vi "Teleop.vi"(10 "Match Info":T1={"Autonomous Elapsed Seconds"=0.0, "TeleOp Elapsed Seconds"=0.0, "Disabled Elapsed Seconds"=0.0, "Visited Autonomous"=FALSE, "Visited TeleOp"=FALSE, "Visited Disabled"=FALSE, "Autonomous Settings"={"Autonomous Style"=enum."Independent", "VI Refnum"=refnum}}, 11 "Call Context":T2) -> ()   [LabVIEW 2013]
doc: "This VI is called for each TeleOp packet received from the DS where the robot is not disabled. It is often used to read from the joysticks and update I/O or to update setpoints for timed control loops. It should complete and return within 20 milliseconds or it may miss DS packets."
uses:
  <vilib>/Rock Robotics/WPI/DriverStation/WPI_DriverStationDerivedRobotMode.ctl
  <vilib>/Rock Robotics/WPI/DriverStation/WPI_DriverStationMatch Info.ctl
  <vilib>/Rock Robotics/WPI/Solenoid/WPI_SolenoidValue.ctl
  Robot Global Data.vi
  <vilib>/Rock Robotics/WPI/Solenoid/Deprecated/WPI_SolenoidGetBool.vi
  <vilib>/Rock Robotics/WPI/Solenoid/WPI_SolenoidSetEnum.vi
  <vilib>/Rock Robotics/WPI/Joystick/WPI_JoystickGetSetRefNum.vi
  <vilib>/Rock Robotics/WPI/RobotDrive/WPI_RobotDriveGetSetRefNum.vi
panel:
  out "Numeric 1":dbl(slide) scale=0.0..100.0
  out "Boolean 2":bool
  out "Boolean 1":bool
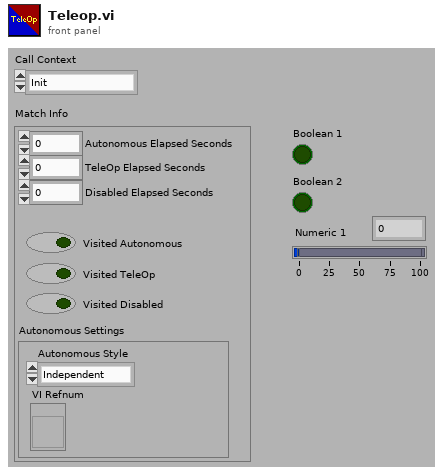
[diagram p1: front panel]
types:
  T1 = typedef "WPI_DriverStationMatch Info.ctl" = cluster{"Autonomous Elapsed Seconds":dbl, "TeleOp Elapsed Seconds":dbl, "Disabled Elapsed Seconds":dbl, "Visited Autonomous":bool, "Visited TeleOp":bool, "Visited Disabled":bool, "Autonomous Settings":cluster{"Autonomous Style":enum16{"Iterative", "Independent"}, "VI Refnum":refnum<vi>}}
  T2 = typedef "WPI_DriverStationDerivedRobotMode.ctl" = enum16{"Init", "Execute", "Stop"}
  T3 = typedef "WPI_JoystickDevRef.ctl" = cluster{"Device":T4}
  T4 = typedef "WPI_JoystickDeviceEnum.ctl" = enum16{"USB 1", "USB 2", "USB 3", "USB 4", "Kinect 1", "Kinect 2"}
  T5 = typedef "WPI_JoystickButtonState.ctl" = cluster{"Button 1":bool, "Button 2":bool, "Button 3":bool, "Button 4":bool, "Button 5":bool, "Button 6":bool, "Button 7":bool, "Button 8":bool, "Button 9":bool, "Button 10":bool, "Button 11":bool, "Button 12":bool}
  T6 = typedef "WPI_SolenoidDevRef.ctl" = cluster{"DevStatus":errorcluster, "Solenoid Module":T7, "Forward Solenoid Channel":T8, "Reverse Solenoid Channel":T8}
  T7 = typedef "FPGA_TypedefSolenoidModule.ctl" = enum16{"Solenoid Module 1", "Solenoid Module 2"}
  T8 = typedef "WPI_SolenoidChannel.ctl" = enum8{"Solenoid 1", "Solenoid 2", "Solenoid 3", "Solenoid 4", "Solenoid 5", "Solenoid 6", "Solenoid 7", "Solenoid 8", "Invalid"}
  T9 = typedef "WPI_SolenoidValue.ctl" = enum16{"Off", "On", "Forward", "Reverse"}
  T10 = typedef "WPI_MotorControlDeviceRef.ctl" = cluster{"DeviceStatus":errorcluster, "Type":enum16{"PWM", "CAN"}, "PWM":cluster{"Digital Module":T11, "PWM Channel":T12, "DeadBand":T13}, "CAN":cluster{"Device Number":u8, "Control Mode":T14, "Semaphore":T15, "Max Vout":dbl}, "Invert":bool, "TransformRef":T16, "InvTransformRef":T16}
  T11 = typedef "FPGA_TypedefDigitalModule.ctl" = enum16{"Digital Module 1", "Digital Module 2"}
  T12 = typedef "FPGA_DIOPWMChannel.ctl" = enum8{"PWM 1", "PWM 2", "PWM 3", "PWM 4", "PWM 5", "PWM 6", "PWM 7", "PWM 8", "PWM 9", "PWM 10", "Invalid"}
  T13 = typedef "WPI_PWMDeadband.ctl" = cluster{"Name":string, "maxPositivePwm":i32, "minPositivePwm":i32, "centerPwm":i32, "maxNegativePwm":i32, "minNegativePwm":i32, "angularRange":u16}
  T14 = typedef "WPI_CANJaguar_ControlMode.ctl" = enum8{"Percent VBus", "Current", "Speed", "Position", "Voltage"}
  T15 = typedef "Semaphore RefNum" = refnum<k1>
  T16 = typedef "WPI_PWMTransform_ConPane.ctl" = refnum<vi>
  T17 = typedef "WPI_RobotDriveDevRef.ctl" = cluster{"DevStatus":errorcluster, "Motors[]":T10[], "Square Inputs":bool, "Max Output":dbl, "Isochronous":bool}
  T18 = cluster{"axis 1 (x)":dbl, "axis 2 (y)":dbl, "axis 3 (throttle)":dbl, "axis 4":dbl, "axis 5":dbl, "axis 6":dbl}
  T19 = typedef "WPI_RelayDevRef.ctl" = cluster{"DevStatus":errorcluster, "Relay Channel":T20, "Digital Module":T11, "Relay Direction":T21}
  T20 = typedef "FPGA_DIORelayChannel.ctl" = enum8{"Relay 1", "Relay 2", "Relay 3", "Relay 4", "Relay 5", "Relay 6", "Relay 7", "Relay 8", "Invalid"}
  T21 = typedef "WPI_RelayDirection.ctl" = enum16{"Both directions", "Forward only", "Reverse only"}
  T22 = typedef "WPI_DigitalInputDevRef.ctl" = cluster{"DevStatus":errorcluster, "DIO Channel":T23, "Digital Module":T11}
  T23 = typedef "FPGA_DIOChannel.ctl" = enum8{"DIO 1", "DIO 2", "DIO 3", "DIO 4", "DIO 5", "DIO 6", "DIO 7", "DIO 8", "DIO 9", "DIO 10", "DIO 11", "DIO 12", "DIO 13", "DIO 14", "Invalid"}
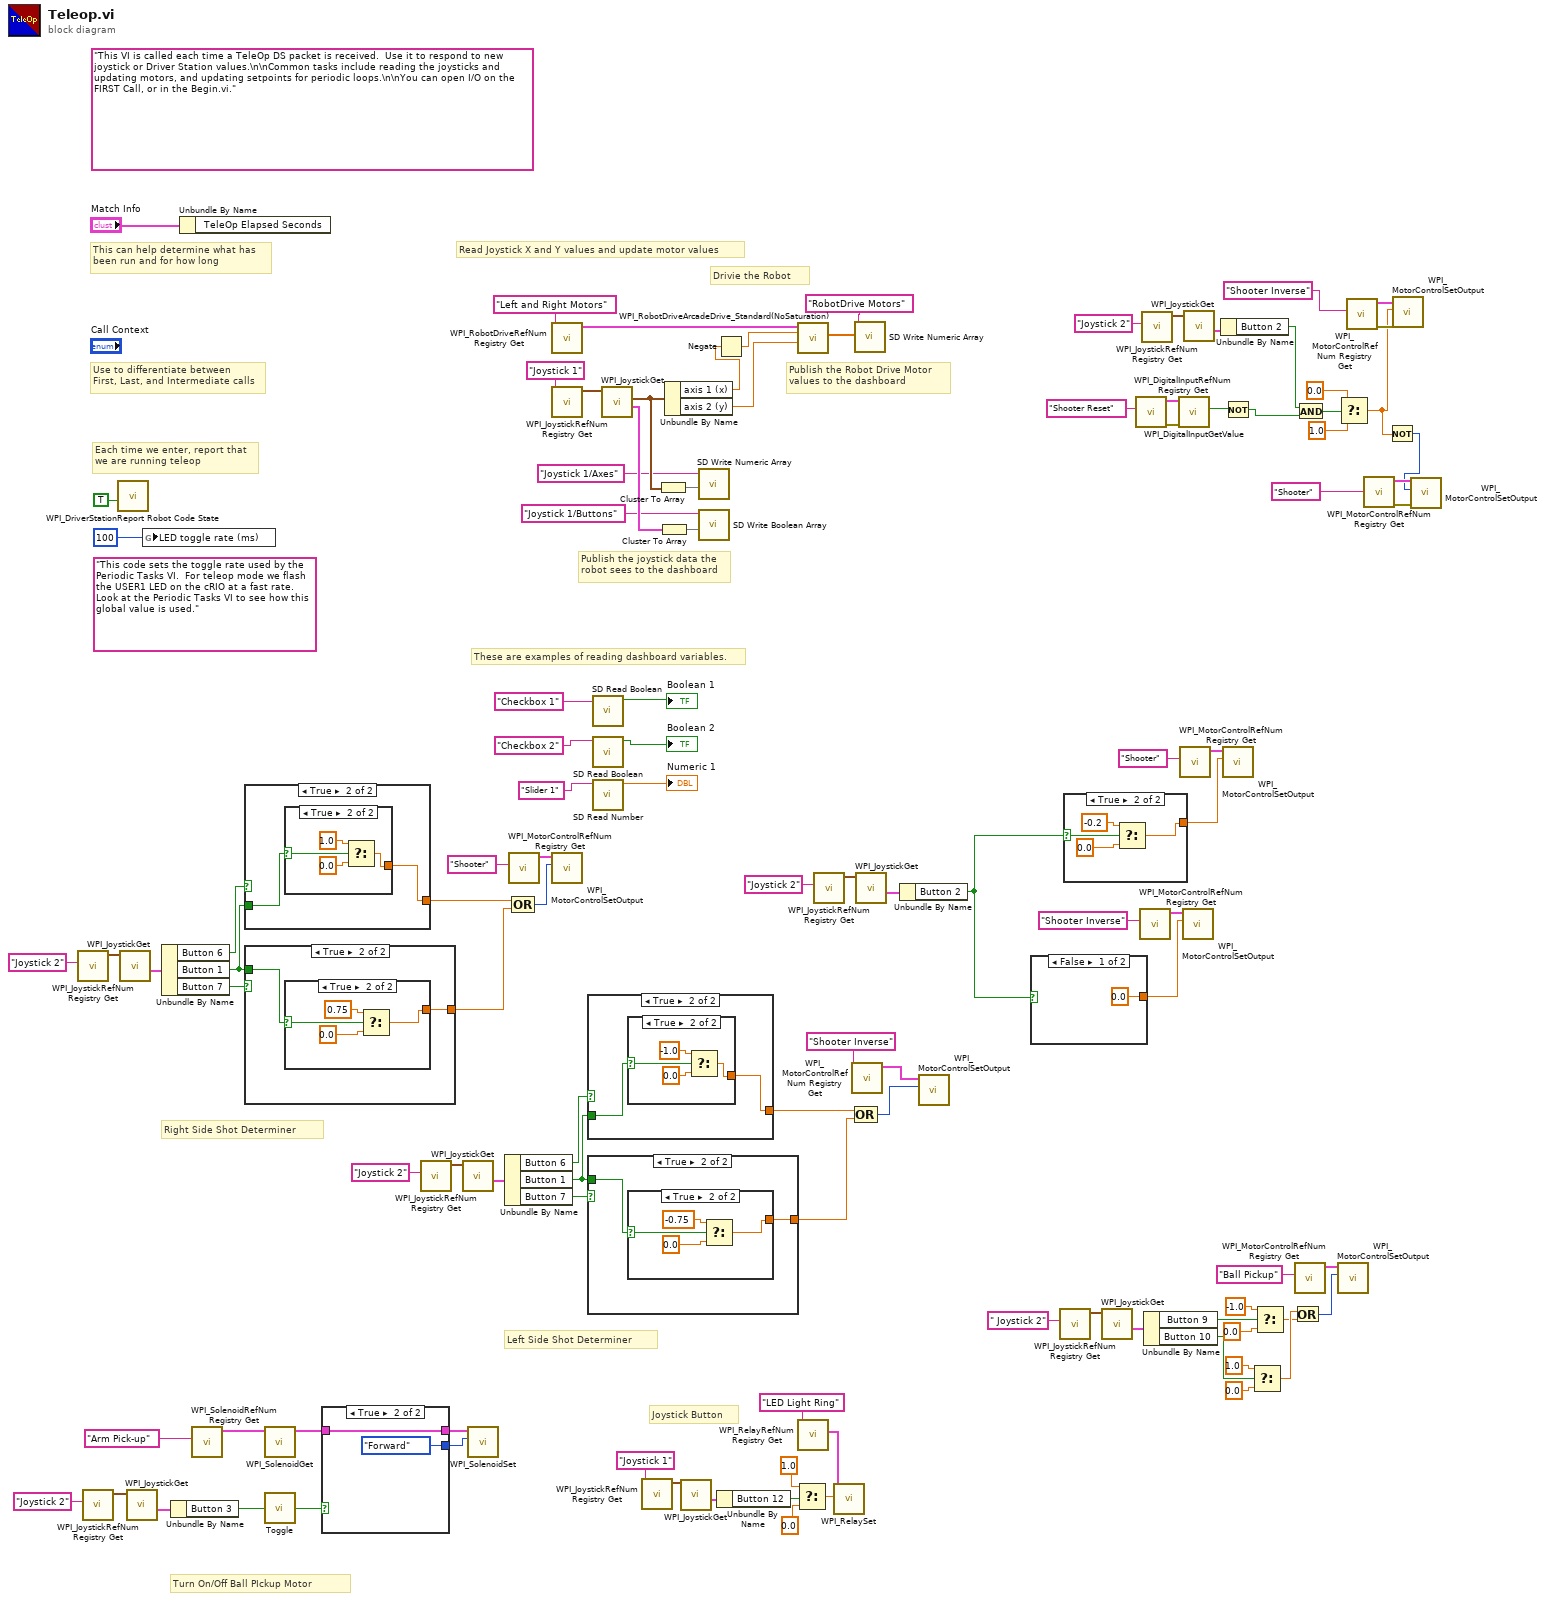
[diagram p0: block diagram]
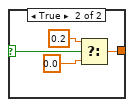
[diagram p2: hidden frame]
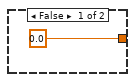
[diagram p3: hidden frame]
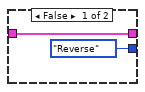
[diagram p4: hidden frame]
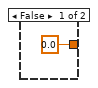
[diagram p5: hidden frame]
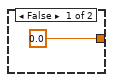
[diagram p6: hidden frame]
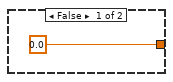
[diagram p7: hidden frame]
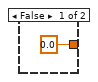
[diagram p8: hidden frame]
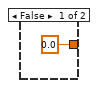
[diagram p9: hidden frame]
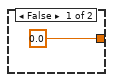
[diagram p10: hidden frame]
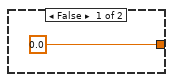
[diagram p11: hidden frame]
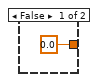
[diagram p12: hidden frame]
diagram:
  (unwired) "This code sets the toggle rate used by the Periodic Tasks VI.  For teleop mode we flash the USER1 LED on the cRIO at a fast rate.  Look at the Periodic Tasks VI to see how this global value is used."
  (unwired) "This VI is called each time a TeleOp DS packet is received.  Use it to respond to new joystick or Driver Station values.\n\nCommon tasks include reading the joysticks and updating motors, and updating setpoints for periodic loops.\n\nYou can open I/O on the FIRST Call, or in the Begin.vi."
  # "Left Side Shot Determiner"
  # "Turn On/Off Ball PIckup Motor"
  # "Right Side Shot Determiner"
  # "Joystick Button"
  # "Drivie the Robot"
  # "These are examples of reading dashboard variables."
  # "Publish the Robot Drive Motor\nvalues to the dashboard"
  # "Publish the joystick data the\nrobot sees to the dashboard"
  # "Each time we enter, report that\nwe are running teleop"
  # "Use to differentiate between\nFirst, Last, and Intermediate calls"
  # "This can help determine what has\nbeen run and for how long"
  # "Read Joystick X and Y values and update motor values"
  n1 = call <vilib>:"WPI_JoystickRefNum Registry Get.vi"("refnum name"="Joystick 2") -> ("JoystickDevRef"=w77:T3)  [unwired: 9 in, 1 out]
  n2 = call <vilib>:"WPI_JoystickRefNum Registry Get.vi"("refnum name"="Joystick 2") -> ("JoystickDevRef"=w71:T3)  [unwired: 9 in, 1 out]
  n3 = call <vilib>:"WPI_DriverStationReport Robot Code State.vi"("TeleOp"=TRUE ("Autonomous")) -> ()  [unwired: 10 in, 1 out]
  n4 = call <vilib>:"WPI_JoystickGet.vi"("JoystickDevRef"=w77) -> ("Buttons"=w76:T5)  [unwired: 4 in, 2 out]
  n5 = call <vilib>:"WPI_JoystickGet.vi"("JoystickDevRef"=w71) -> ("Buttons"=w70:T5)  [unwired: 4 in, 2 out]
  n6 = global write "Robot Global Data.vi" "LED toggle rate (ms)"(u32 100 ("LED ms toggle rate")) -> ()
  n7 = Unbundle By Name(w76) -> ("Button 6"=w66:bool, "Button 1"=w64:bool, "Button 7"=w65:bool)
  n8 = Unbundle By Name(w70) -> ("Button 3"=w67:bool)
  n9 = Unbundle By Name("Match Info") -> ()  [unwired: 1 out]
  n10 = call <vilib>:"WPI_SolenoidRefNum Registry Get.vi"("refnum name"="Arm Pick-up") -> ("SolenoidDevRef"=w35:T6)  [unwired: 9 in, 1 out]
  n11 = case shown="True" w66 {
    tunnel: w64 -> [_ w112]
    tunnel: [0.0 ("f") w111] -> w63
    frame False {
    }
    frame True {
      n12 = case shown="True" w112 {
        selector: w112 -> [_ w115]
        tunnel: [0.0 ("f") w114] -> w111
        frame False {
        }
        frame True {
          n13 = Select(t=1.0, s=w115, f=0.0) -> (s? t:f=w114:dbl)
        }
      }
    }
  }
  n14 = case shown="True" w65 {
    tunnel: w64 -> [_ w120]
    tunnel: [0.0 ("f") w119] -> w62
    frame False {
    }
    frame True {
      n15 = case shown="True" w120 {
        selector: w120 -> [_ w123]
        tunnel: [0.0 ("f") w122] -> w119
        frame False {
        }
        frame True {
          n16 = Select(t=0.75, s=w123, f=0.0) -> (s? t:f=w122:dbl)
        }
      }
    }
  }
  n17 = call-poly <vilib>:"WPI_SolenoidGet.vi"("SolenoidDevRef"=w35) -> ("SolenoidDevRef"=w33:T6)  [unwired: 8 in, 2 out]
  n18 = call "Toggle.vi"("Input"=w67) -> ("Toggled Output"=w34:bool)
  n19 = case shown="True" w34 {
    tunnel: w33 -> [w127 w129]
    tunnel: [w127 w129] -> w32
    tunnel: [WPI_SolenoidValue."Reverse" ("Value") WPI_SolenoidValue."Forward" ("Value")] -> w31
    frame False {
    }
    frame True {
    }
  }
  n20 = call <vilib>:"WPI_JoystickRefNum Registry Get.vi"("refnum name"="Joystick 2") -> ("JoystickDevRef"=w49:T3)  [unwired: 9 in, 1 out]
  n21 = call <vilib>:"WPI_JoystickGet.vi"("JoystickDevRef"=w49) -> ("Buttons"=w50:T5)  [unwired: 4 in, 2 out]
  n22 = call-poly <vilib>:"WPI_SolenoidSet.vi"("Value"=w31, "SolenoidDevRef"=w32) -> ()  [unwired: 8 in, 2 out]
  n23 = Unbundle By Name(w50) -> ("Button 6"=w51:bool, "Button 1"=w53:bool, "Button 7"=w52:bool)
  n24 = call <vilib>:"WPI_MotorControlRefNum Registry Get.vi"("refnum name"="Shooter") -> ("MotorControlDevRef"=w59:T10)  [unwired: 9 in, 1 out]
  n25 = Compound Arithmetic op=OR(w63, w62) -> (w61:i32)
  n26 = call <vilib>:"WPI_RobotDriveRefNum Registry Get.vi"("refnum name"="Left and Right Motors") -> ("RobotDriveDevRef"=w107:T17)  [unwired: 1 in, 9 out]
  n27 = call <vilib>:"WPI_JoystickRefNum Registry Get.vi"("refnum name"="Joystick 1") -> ("JoystickDevRef"=w104:T3)  [unwired: 1 in, 9 out]
  n28 = call <vilib>:"WPI_MotorControlSetOutput.vi"("Output"=w61, "MotorControlDevRef"=w59) -> ()  [unwired: 7 in, 3 out]
  n29 = case shown="True" w51 {
    tunnel: w53 -> [_ w132]
    tunnel: [0.0 ("f") w131] -> w54
    frame False {
    }
    frame True {
      n30 = case shown="True" w132 {
        selector: w132 -> [_ w135]
        tunnel: [0.0 ("f") w134] -> w131
        frame False {
        }
        frame True {
          n31 = Select(t=-1.0, s=w135, f=0.0) -> (s? t:f=w134:dbl)
        }
      }
    }
  }
  n32 = case shown="True" w52 {
    tunnel: w53 -> [_ w140]
    tunnel: [0.0 ("f") w139] -> w55
    frame False {
    }
    frame True {
      n33 = case shown="True" w140 {
        selector: w140 -> [_ w143]
        tunnel: [0.0 ("f") w142] -> w139
        frame False {
        }
        frame True {
          n34 = Select(t=-0.75, s=w143, f=0.0) -> (s? t:f=w142:dbl)
        }
      }
    }
  }
  n35 = call <vilib>:"SD Read Boolean.vi"("Name"="Checkbox 1" ("refnum name")) -> ("Boolean"=→"Boolean 1":bool)  [unwired: 8 in, 2 out]
  n36 = call <vilib>:"SD Read Boolean.vi"("Name"="Checkbox 2" ("refnum name")) -> ("Boolean"=→"Boolean 2":bool)  [unwired: 8 in, 2 out]
  n37 = call <vilib>:"SD Read Number.vi"("Name"="Slider 1" ("refnum name")) -> ("Numeric"=→"Numeric 1":dbl)  [unwired: 8 in, 2 out]
  n38 = call <vilib>:"WPI_JoystickGet.vi"("JoystickDevRef"=w104) -> ("Buttons"=w101:T5, "Axes"=w98:T18)  [unwired: 1 in, 4 out]
  n39 = call <vilib>:"WPI_JoystickRefNum Registry Get.vi"("refnum name"="Joystick 1") -> ("JoystickDevRef"=w83:T3)  [unwired: 9 in, 1 out]
  n40 = Cluster To Array(cluster=w98) -> (array=w97:dbl[])
  n41 = Cluster To Array(cluster=w101) -> (array=w100:bool[])
  n42 = Unbundle By Name(w98) -> ("axis 1 (x)"=w69:dbl, "axis 2 (y)"=w106:dbl)
  n43 = call <vilib>:"WPI_JoystickGet.vi"("JoystickDevRef"=w83) -> ("Buttons"=w82:T5)  [unwired: 4 in, 2 out]
  n44 = call <vilib>:"SD Write Numeric Array.vi"("Numeric Array"=w97, "Name"="Joystick 1/Axes") -> ()  [unwired: 8 in, 2 out]
  n45 = call <vilib>:"SD Write Boolean Array.vi"("Boolean Array"=w100, "Name"="Joystick 1/Buttons") -> ()  [unwired: 8 in, 2 out]
  n46 = Negate(x=w69) -> (-x=w68:dbl)
  n47 = Unbundle By Name(w82) -> ("Button 12"=w81:bool)
  n48 = Select(t=1.0, s=w81, f=0.0) -> (s? t:f=w80:dbl)
  n49 = call <vilib>:"WPI_RobotDriveArcadeDrive_Standard(NoSaturation).vi"("Y axis value"=w106, "X axis value"=w68, "RobotDriveDevRef"=w107) -> ("Motor Values"=w94:dbl[])  [unwired: 1 in, 7 out]
  n50 = call <vilib>:"WPI_RelayRefNum Registry Get.vi"("refnum name"="LED Light Ring") -> ("RelayDevRef"=w87:T19)  [unwired: 9 in, 1 out]
  n51 = call <vilib>:"WPI_JoystickRefNum Registry Get.vi"("refnum name"="Joystick 2") -> ("JoystickDevRef"=w29:T3)  [unwired: 9 in, 1 out]
  n52 = call <vilib>:"WPI_RelaySet.vi"("RelayValue"=w80, "RelayDevRef"=w87) -> ()  [unwired: 8 in, 2 out]
  n53 = call <vilib>:"WPI_MotorControlRefNum Registry Get.vi"("refnum name"="Shooter Inverse") -> ("MotorControlDevRef"=w58:T10)  [unwired: 9 in, 1 out]
  n54 = call <vilib>:"SD Write Numeric Array.vi"("Numeric Array"=w94, "Name"="RobotDrive Motors") -> ()  [unwired: 8 in, 2 out]
  n55 = Compound Arithmetic op=OR(w54, w55) -> (w56:i32)
  n56 = call <vilib>:"WPI_JoystickGet.vi"("JoystickDevRef"=w29) -> ("Buttons"=w28:T5)  [unwired: 4 in, 2 out]
  n57 = Unbundle By Name(w28) -> ("Button 2"=w27:bool)
  n58 = call <vilib>:"WPI_MotorControlSetOutput.vi"("Output"=w56, "MotorControlDevRef"=w58) -> ()  [unwired: 7 in, 3 out]
  n59 = case shown="False" w27 {
    selector: w27 -> [_ w150]
    tunnel: [0.0 ("f") w147] -> w24
    frame False {
    }
    frame True {
      n60 = Select(t=0.2, s=w150, f=0.0) -> (s? t:f=w147:dbl)
    }
  }
  n61 = call <vilib>:"WPI_JoystickRefNum Registry Get.vi"("refnum name"=" Joystick 2") -> ("JoystickDevRef"=w41:T3)  [unwired: 9 in, 1 out]
  n62 = case shown="True" w27 {
    selector: w27 -> [_ w155]
    tunnel: [0.0 ("f") w152] -> w21
    frame False {
    }
    frame True {
      n63 = Select(t=-0.2, s=w155, f=0.0) -> (s? t:f=w152:dbl)
    }
  }
  n64 = call <vilib>:"WPI_JoystickGet.vi"("JoystickDevRef"=w41) -> ("Buttons"=w42:T5)  [unwired: 4 in, 2 out]
  n65 = call <vilib>:"WPI_DigitalInputRefNum Registry Get.vi"("refnum name"="Shooter Reset") -> ("error out"=w16:errorcluster, "DigitalInputDevRef"=w15:T22)  [unwired: 9 in]
  n66 = call <vilib>:"WPI_MotorControlRefNum Registry Get.vi"("refnum name"="Shooter Inverse") -> ("MotorControlDevRef"=w25:T10)  [unwired: 9 in, 1 out]
  n67 = call <vilib>:"WPI_JoystickRefNum Registry Get.vi"("refnum name"="Joystick 2") -> ("JoystickDevRef"=w19:T3)  [unwired: 9 in, 1 out]
  n68 = Unbundle By Name(w42) -> ("Button 9"=w43:bool, "Button 10"=w39:bool)
  n69 = call <vilib>:"WPI_DigitalInputGetValue.vi"("error in (no error)"=w16, "DigitalInputDevRef"=w15) -> ("Value"=w14:bool)  [unwired: 7 in, 2 out]
  n70 = call <vilib>:"WPI_MotorControlRefNum Registry Get.vi"("refnum name"="Shooter") -> ("MotorControlDevRef"=w23:T10)  [unwired: 9 in, 1 out]
  n71 = call <vilib>:"WPI_MotorControlSetOutput.vi"("Output"=w24, "MotorControlDevRef"=w25) -> ()  [unwired: 7 in, 3 out]
  n72 = call <vilib>:"WPI_JoystickGet.vi"("JoystickDevRef"=w19) -> ("Buttons"=w18:T5)  [unwired: 4 in, 2 out]
  n73 = Unbundle By Name(w18) -> ("Button 2"=w12:bool)
  n74 = Not(x=w14) -> (.not. x?=w13:bool)
  n75 = call <vilib>:"WPI_MotorControlSetOutput.vi"("Output"=w21, "MotorControlDevRef"=w23) -> ()  [unwired: 7 in, 3 out]
  n76 = Select(t=1.0, s=w39, f=0.0) -> (s? t:f=w38:dbl)
  n77 = Select(t=-1.0, s=w43, f=0.0) -> (s? t:f=w37:dbl)
  n78 = Or(x=w38, y=w37) -> (x .or. y?=w36:i32)
  n79 = call <vilib>:"WPI_MotorControlRefNum Registry Get.vi"("refnum name"="Ball Pickup") -> ("MotorControlDevRef"=w74:T10)  [unwired: 9 in, 1 out]
  n80 = And(x=w12, y=w13) -> (x .and. y?=w9:bool)
  n81 = call <vilib>:"WPI_MotorControlSetOutput.vi"("Output"=w36, "MotorControlDevRef"=w74) -> ()  [unwired: 7 in, 3 out]
  n82 = Select(t=0.0, s=w9, f=1.0) -> (s? t:f=w4:dbl)
  n83 = call <vilib>:"WPI_MotorControlRefNum Registry Get.vi"("refnum name"="Shooter Inverse") -> ("error out"=w11:errorcluster, "MotorControlDevRef"=w10:T10)  [unwired: 9 in]
  n84 = call <vilib>:"WPI_MotorControlRefNum Registry Get.vi"("refnum name"="Shooter") -> ("error out"=w6:errorcluster, "MotorControlDevRef"=w5:T10)  [unwired: 9 in]
  n85 = Not(x=w4) -> (.not. x?=w3:u32)
  n86 = call <vilib>:"WPI_MotorControlSetOutput.vi"("error in (no error)"=w11, "Output"=w4, "MotorControlDevRef"=w10) -> ()  [unwired: 6 in, 3 out]
  n87 = call <vilib>:"WPI_MotorControlSetOutput.vi"("error in (no error)"=w6, "Output"=w3, "MotorControlDevRef"=w5) -> ()  [unwired: 6 in, 3 out]
